vi "HB_Simple.appendData2Variant.vi"(0 "initData":variant, 2 "x":dbl, 3 "statusEvent":refnum<class "HGF_TriggeredEvent.lvclass">, 4 "publish_X":refnum<class "HGF_PVPublisher.lvclass">, 5 "error in (no error)":errorcluster) -> (14 "dup initData":variant, 19 "error out":errorcluster)   [LabVIEW 2009, in "HB_BaseClass_Examples.lvlib" / "HB_Simple.lvclass"]
doc: "Append initialize data to variant."
uses:
  HB_Simple.lvclass
  lib.lib/HGF_LVC/HGF_BaseClasses/HGF_TriggeredEvent/HGF_TriggeredEvent.lvclass
  lib.lib/HGF_LVC/HGF_BaseClasses/HGF_PVPublisher/HGF_PVPublisher.lvclass
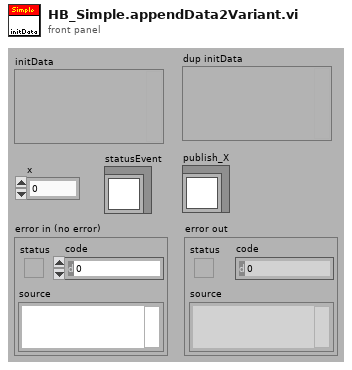
[diagram p1: front panel]
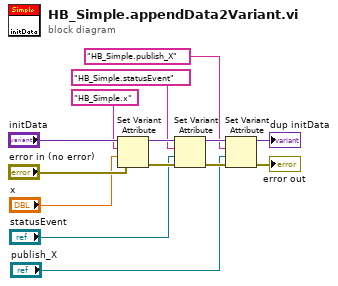
[diagram p0: block diagram]
diagram:
  n1 = Set Variant Attribute(Variant="initData", name="HB_Simple.x", value="x", error in="error in (no error)") -> (Variant out=w10:variant, error out=w9:errorcluster)  [unwired: 1 out]
  n2 = Set Variant Attribute(Variant=w10, name="HB_Simple.statusEvent", value="statusEvent", error in=w9) -> (Variant out=w6:variant, error out=w5:errorcluster)  [unwired: 1 out]
  n3 = Set Variant Attribute(Variant=w6, name="HB_Simple.publish_X", value="publish_X", error in=w5) -> (Variant out=→"dup initData":variant, error out=→"error out":errorcluster)  [unwired: 1 out]
